vi "set autostart enable status.vi"(8 "error in (no error)":errorcluster, 11 "Cobolt in":refnum<class "Cobolt.lvclass">) -> (0 "error out":errorcluster, 3 "Cobolt out":refnum<class "Cobolt.lvclass">)   [LabVIEW 2012, in "Cobolt.lvclass"]
uses:
  Cobolt.lvclass
  CoboltLaserDrivers_Public_LV2012/CoboltLaser_Controls/ExpectedResponseType.ctl
  Cobolt.lvclass/Cobolt.ctl
panel:
  out "buffer out":string
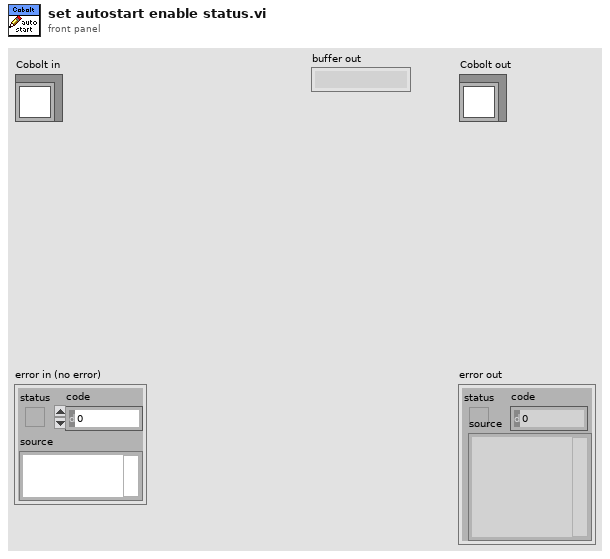
[diagram p1: front panel]
types:
  T1 = typedef "Cobolt.lvclass/ExpectedResponseType.ctl" = u16
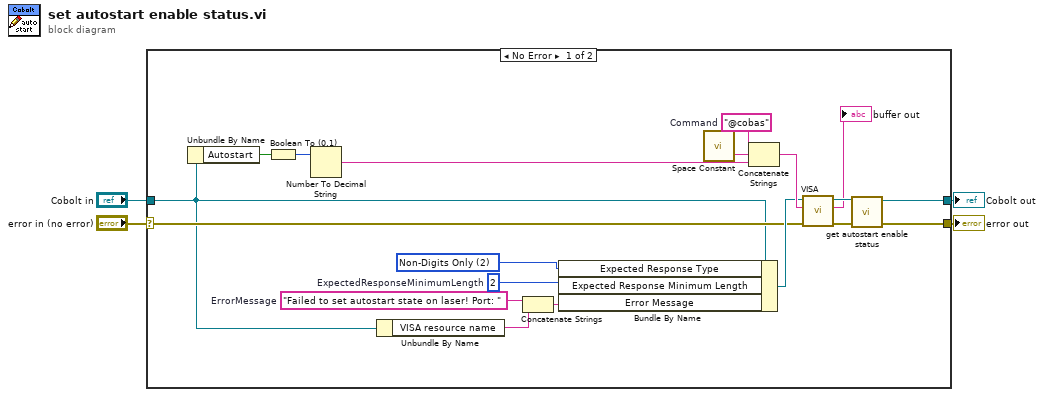
[diagram p0: block diagram]
diagram:
  n1 = case shown="No Error" "error in (no error)" {
    selector: "error in (no error)" -> [w12 w25]
    tunnel: [w11 w25] -> w3
    tunnel: [w8 w24] -> w1
    tunnel: "Cobolt in" -> [w9 w24]
    frame No Error {
      w14 = T1 2 items=["Any", "Digits Only", "Non-Digits Only"] ("ExpectedResponseType")
      w18 = 2  # ExpectedResponseMinimumLength
      w16 = "Failed to set autostart state on laser! Port: "  # ErrorMessage
      w7 = "@cobas"  # Command
      n2 = Unbundle By Name(w9) -> ("Autostart"=w20:bool)
      n3 = Boolean To (0,1)(Boolean=w20) -> (0, 1=w21:i16)
      n4 = Number To Decimal String(number=w21) -> (decimal integer string=w22:string)  [unwired: 1 in]
      n5 = Unbundle By Name(w9) -> ("VISA resource name"=w17:string)
      n6 = Concatenate Strings(w16, w17) -> (w15:string)
      n7 = Bundle By Name(cluster=w9, "Expected Response Type"=w14, "Expected Response Minimum Length"=w18, "Error Message"=w15) -> (w19:refnum<class "Cobolt.lvclass">)
      n8 = call <vilib>:"Space Constant.vi"() -> ("String"=w6:string)
      n9 = Concatenate Strings(w7, w6, w22) -> (w23:string)
      n10 = call-dynamic "VISA.vi"("error in (no error)"=w12, "string to write"=w23, "Cobolt in"=w19) -> ("error out"=w13:errorcluster, "buffer out"=→"buffer out":string, "Cobolt out"=w10:refnum<class "Cobolt.lvclass">)  [unwired: 6 in]
      n11 = call-dynamic "get autostart enable status.vi"("error in (no error)"=w13, "Cobolt in"=w10) -> ("error out"=w11:errorcluster, "Cobolt out"=w8:refnum<class "Cobolt.lvclass">)  [unwired: 8 in]
    }
    frame Error {
    }
  }
  "error out" <- w3
  "Cobolt out" <- w1
